vi "XYStage.GetPosition.vi"(8 "error in (no error)":errorcluster, 11 "XYStage.KIM101 in":refnum<class "XYStage.KIM101.lvclass">) -> (0 "error out":errorcluster, 2 "Coordinates":T1, 3 "XYStage.KIM101 out":refnum<class "XYStage.KIM101.lvclass">)   [LabVIEW 2017, in "XYStage.KIM101.lvclass"]
uses:
  XYStage.KIM101.lvclass
  D:/upwork/Laser Measurement Tool/Laser/project/Subsystems/XYStage/XYStage.lvclass
  XYStage/Typedefs/Coordinates--Cluster.ctl
  XYStage/Typedefs/Coordinates.Units--Cluster.ctl
  XYStage/Typedefs/Coordinates.Counts--Cluster.ctl
  D:/upwork/Laser Measurement Tool/Laser/project/data/Thorlabs.MotionControl.KCube.InertialMotorCLI.dll
  data/Thorlabs.MotionControl.KCube.InertialMotorCLI.dll
  XYStage/XYStage.lvclass
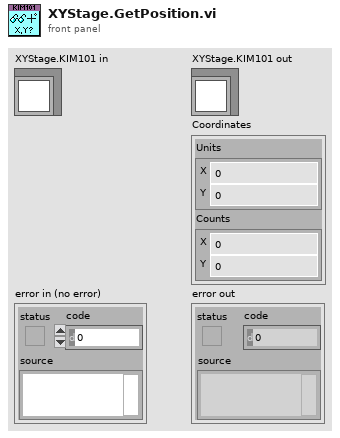
[diagram p1: front panel]
types:
  T1 = typedef "XYStage.lvclass/Coordinates--Cluster.ctl" = cluster{"Units":T2, "Counts":T3}
  T2 = typedef "XYStage.lvclass/Coordinates.Units--Cluster.ctl" = cluster{"X":dbl, "Y":dbl}
  T3 = typedef "XYStage.lvclass/Coordinates.Counts--Cluster.ctl" = cluster{"X":i32, "Y":i32}
  T4 = typedef "XYStage.KIM101.lvclass/Resource--Cluster.ctl" = cluster{"KCubeInertialMotorControl":refnum<k24>, "Device":refnum<k24>, "X Axis Channel":i32, "Y Axis Channel":i32}
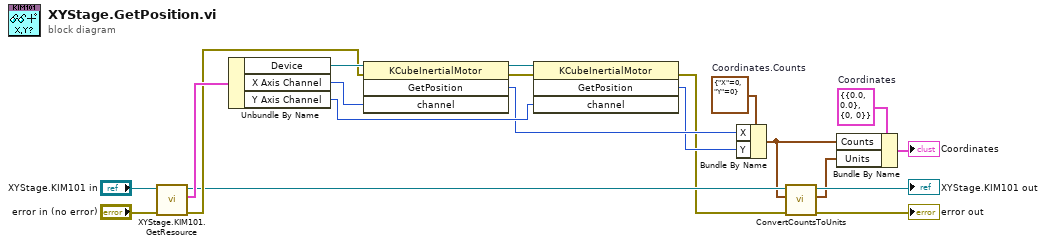
[diagram p0: block diagram]
diagram:
  w7 = T1 {"Units"={"X"=0.0, "Y"=0.0}, "Counts"={"X"=0, "Y"=0}}  # Coordinates
  w11 = T3 {"X"=0, "Y"=0}  # Coordinates.Counts
  n1 = call "XYStage.KIM101.GetResource.vi"("error in (no error)"="error in (no error)", "XYStage.KIM101 in"="XYStage.KIM101 in") -> ("error out"=w15:errorcluster, "Resource"=w18:T4, "XYStage.KIM101 out"=w6:refnum<class "XYStage.KIM101.lvclass">)  [unwired: 7 in]
  n2 = Unbundle By Name(w18) -> ("Device"=w17:refnum<k24>, "X Axis Channel"=w16:i32, "Y Axis Channel"=w12:i32)
  n3 = invoke class="KCubeInertialMotor" method="GetPosition"(reference=w17, error in=w15, "channel"=w16) -> (reference out=w14:refnum<k24>, error out=w13:errorcluster, "GetPosition"=w10:i32)  [unwired: 1 in, 1 out]
  n4 = invoke class="KCubeInertialMotor" method="GetPosition"(reference=w14, error in=w13, "channel"=w12) -> (error out=w2:errorcluster, "GetPosition"=w9:i32)  [unwired: 1 in, 2 out]
  n5 = Bundle By Name(cluster=w11, "X"=w10, "Y"=w9) -> (w3:T3)
  n6 = call "ConvertCountsToUnits.vi"("error in (no error)"=w2, "Coordinates.Counts"=w3, "XYStage in"=w6) -> ("error out"=→"error out":errorcluster, "Coordinates.Units"=w4:T2, "XYStage out"=→"XYStage.KIM101 out":refnum<class "XYStage.KIM101.lvclass">)  [unwired: 6 in]
  n7 = Bundle By Name(cluster=w7, "Counts"=w3, "Units"=w4) -> (→"Coordinates":T1)
